vi "FEA_Model_Setter.vi"(8 "error in (no error)":errorcluster, 9 "Simulation Parameters input controls":T1, 10 "Modeling Parameters input controls":T2, 11 "FEA_Model in":refnum<class "FEA_Model.lvclass">) -> (0 "error out":errorcluster, 3 "FEA_Model out":refnum<class "FEA_Model.lvclass">)   [LabVIEW 2021, in "FEA_Model.lvclass"]
uses:
  FEA_Model.lvclass
  FEA_Model.lvclass/FEA_Model.ctl
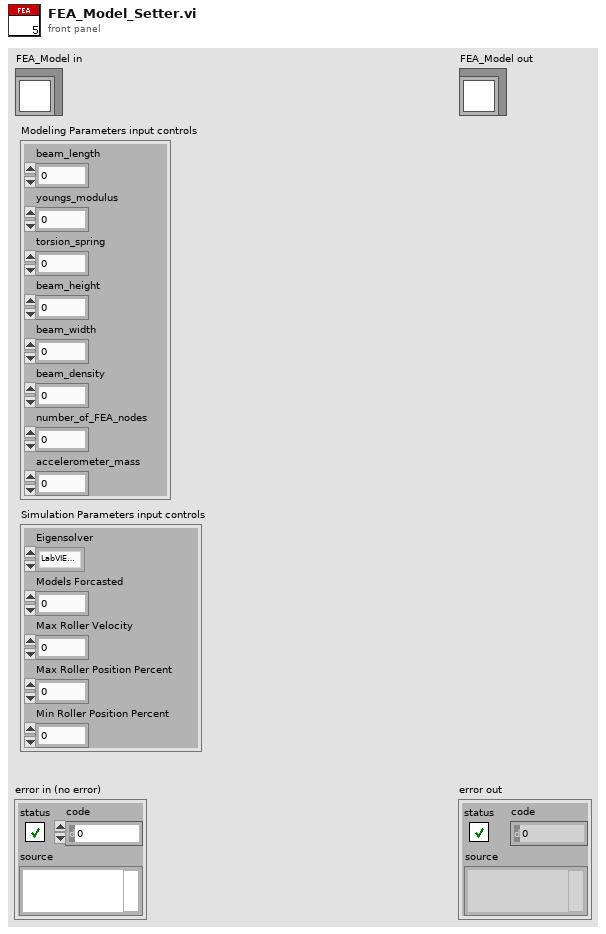
[diagram p1: front panel]
types:
  T1 = cluster{"Eigensolver ":enum16{"LabVIEW Cholesky", "LabVIEW General", "LabVIEW Inverse", "LEMP"}, "Models Forcasted":i32, "Max Roller Velocity":dbl, "Max Roller Position Percent":dbl, "Min Roller Position Percent":dbl}
  T2 = cluster{"beam_length":dbl, "youngs_modulus":dbl, "torsion_spring":dbl, "beam_height":dbl, "beam_width":dbl, "beam_density":dbl, "number_of_FEA_nodes":i32, "accelerometer_mass":dbl}
  T3 = enum16{"LabVIEW Cholesky", "LabVIEW General", "LabVIEW Inverse", "LEMP"}
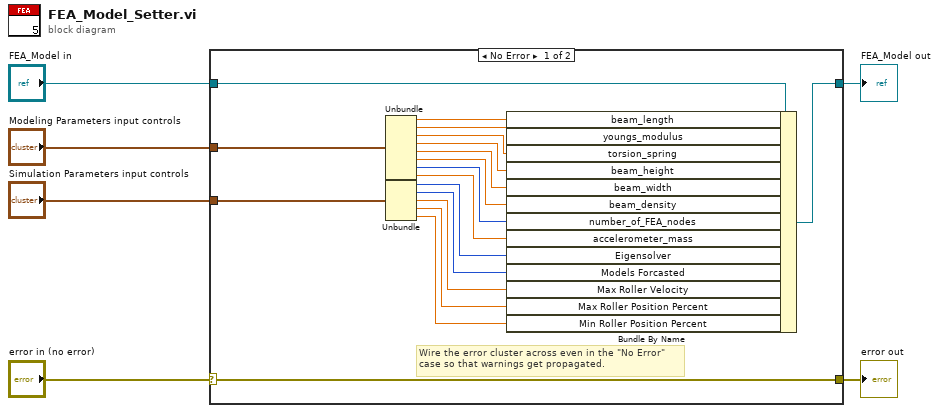
[diagram p0: block diagram]
diagram:
  n1 = case shown="No Error" "error in (no error)" {
    selector: "error in (no error)" -> [w24 w26]
    tunnel: [w24 w26] -> w5
    tunnel: [w22 w25] -> w3
    tunnel: "FEA_Model in" -> [w23 w25]
    tunnel: "Modeling Parameters input controls" -> [w13 _]
    tunnel: "Simulation Parameters input controls" -> [w12 _]
    frame No Error {
      # "Wire the error cluster across even in the \"No Error\"\ncase so that warnings get propagated."
      n2 = Unbundle(w13) -> ("beam_length"=w21:dbl, "youngs_modulus"=w20:dbl, "torsion_spring"=w19:dbl, "beam_height"=w18:dbl, "beam_width"=w17:dbl, "beam_density"=w16:dbl, "number_of_FEA_nodes"=w15:i32, "accelerometer_mass"=w14:dbl)
      n3 = Unbundle(w12) -> ("Eigensolver"=w11:T3, "Models Forcasted"=w10:i32, "Max Roller Velocity"=w9:dbl, "Max Roller Position Percent"=w8:dbl, "Min Roller Position Percent"=w7:dbl)
      n4 = Bundle By Name(cluster=w23, "beam_length"=w21, "youngs_modulus"=w20, "torsion_spring"=w19, "beam_height"=w18, "beam_width"=w17, "beam_density"=w16, "number_of_FEA_nodes"=w15, "accelerometer_mass"=w14, "Eigensolver"=w11, "Models Forcasted"=w10, "Max Roller Velocity"=w9, "Max Roller Position Percent"=w8, "Min Roller Position Percent"=w7) -> (w22:refnum<class "FEA_Model.lvclass">)
    }
    frame Error {
    }
  }
  "error out" <- w5
  "FEA_Model out" <- w3
